vi "TcpDataReceived.vi"(8 "error in (no error)":errorcluster, 10 "DataReceived":refnum<class "DataReceived.lvclass">, 11 "Cli in":refnum<class "Cli.lvclass">) -> (0 "error out":errorcluster, 3 "Cli out":refnum<class "Cli.lvclass">)   [LabVIEW 2022 SP3, in "Cli.lvlib" / "Cli.lvclass"]
uses:
  Cli.lvclass
  Tcp/DataReceived/DataReceived.lvclass
  Cli.lvclass/Cli.ctl
  Tcp/DataReceived/DataReceived.lvclass/DataReceived.ctl
  ArgumentParser/Source/ParsedData/ParsedData.lvclass/ParsedData.ctl
  Tcp/Tcp Messages/ConnectionWriteData Msg/ConnectionWriteData Msg.lvclass/ConnectionWriteData Msg.ctl
  <vilib>/ActorFramework/Message Enqueuer/Message Enqueuer.lvclass/Message Enqueuer.ctl
  Tcp/DataReceived/Read Data.vi
  Tcp/DataReceived/Read Refnum.vi
  ArgumentParser/Source/ParsedData/Read Arguments.vi
  ArgumentParser/Source/ParsedData/Read StdOut.vi
  ArgumentParser/Source/ParsedData/Read StdErr.vi
  <vilib>/ActorFramework/Message Enqueuer/Enqueue.vi
  Tcp/Tcp Messages/ConnectionWriteData Msg/ConnectionWriteData Msg.lvclass
  C:/Program Files (x86)/National Instruments/LabVIEW 2022/vi.lib/ActorFramework/Message/Message.lvclass
  <vilib>/ActorFramework/Message Priority Queue/Priority Enqueue.vi
  ArgumentParser/Source/ArgumentParser/ArgumentParser.lvclass
  Tcp/DataToSend/DataToSend.lvclass
  CommandReceived/CommandReceived.lvclass
  ArgumentParser/Source/ParsedData/ParsedData.lvclass
  <vilib>/ActorFramework/Actor/Actor.lvclass
  CallerMessage Messages/CliCommandReceived Msg/CliCommandReceived Msg.lvclass
  C:/Program Files (x86)/National Instruments/LabVIEW 2022/vi.lib/ActorFramework/Actor/Actor.lvclass
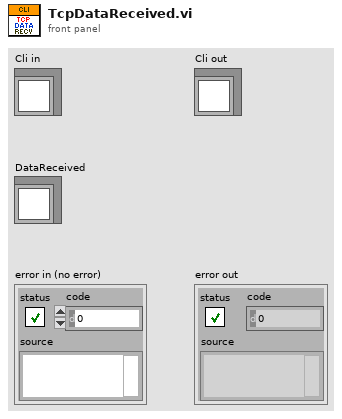
[diagram p1: front panel]
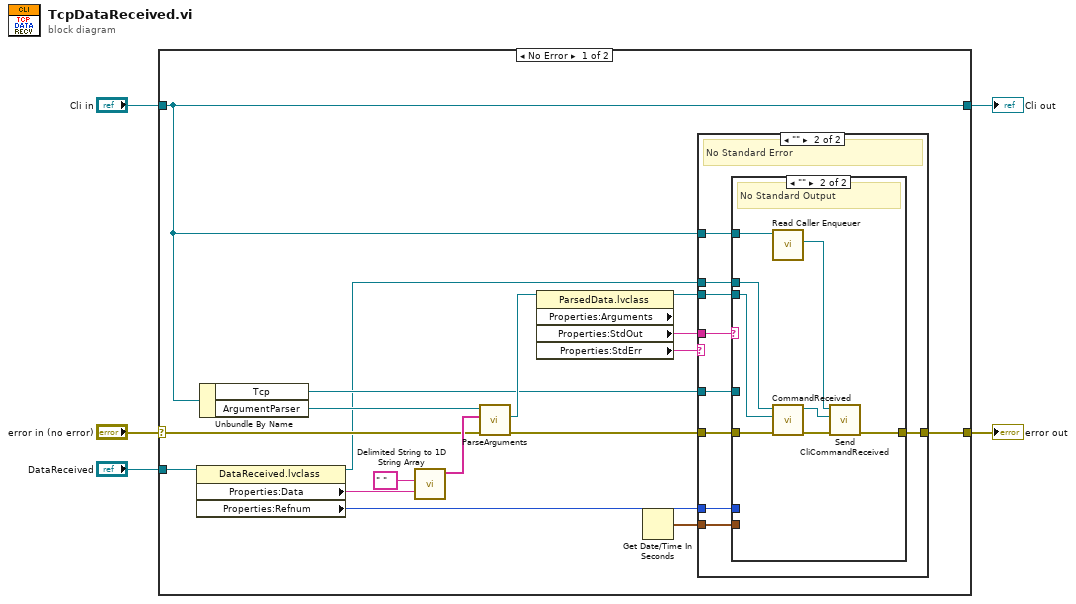
[diagram p0: block diagram]
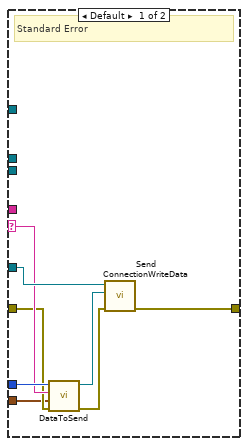
[diagram p2: hidden frame]
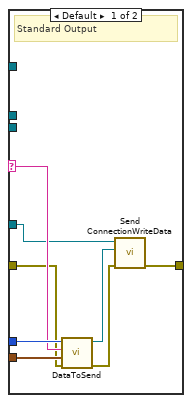
[diagram p3: hidden frame]
diagram:
  n1 = case shown="No Error" "error in (no error)" {
    selector: "error in (no error)" -> [w17 w57]
    tunnel: [w15 w57] -> w2
    tunnel: [w6 w56] -> w1
    tunnel: "Cli in" -> [w6 w56]
    tunnel: "DataReceived" -> [w18 _]
    frame No Error {
      n2 = property class="DataReceived.lvclass"(reference=w18) -> (reference out=w8:refnum<class "DataReceived.lvclass">, "Properties:Data"=w21:string, "Properties:Refnum"=w11:u64)  [unwired: 1 in, 1 out]
      n3 = Unbundle By Name(w6) -> ("Tcp"=w12:refnum<class "Message Enqueuer.lvclass">, "ArgumentParser"=w19:refnum<class "ArgumentParser.lvclass">)
      n4 = call <vilib>:"Delimited String to 1D String Array.vi"("delimiter"=" ", "delimited string"=w21) -> ("string array"=w20:string[])  [unwired: 9 in]
      n5 = call-dynamic "ParseArguments.vi"("error in (no error)"=w17, "CliArguments"=w20, "ArgumentParser in"=w19) -> ("error out"=w14:errorcluster, "ParsedData"=w16:refnum<class "ParsedData.lvclass">)  [unwired: 6 in, 1 out]
      n6 = property class="ParsedData.lvclass" props=["Properties:Arguments", "Properties:StdOut", "Properties:StdErr"](reference=w16) -> (reference out=w7:refnum<class "ParsedData.lvclass">, "Properties:StdOut"=w10:string, "Properties:StdErr"=w13:string)  [unwired: 1 in, 2 out]
      n7 = Get Date/Time In Seconds() -> (seconds since 1Jan1904=w9:timestamp)
      n8 = case shown="\"\"" w13 {
        selector: w13 -> [w27 _]
        tunnel: [w30 w38] -> w15
        tunnel: w14 -> [w25 w37]
        tunnel: w12 -> [w29 w34]
        tunnel: w11 -> [w28 w36]
        tunnel: w10 -> [_ w39]
        tunnel: w9 -> [w23 w35]
        tunnel: w8 -> [_ w33]
        tunnel: w7 -> [_ w32]
        tunnel: w6 -> [_ w31]
        frame Default {
          # "Standard Error"
          n9 = call "DataToSend.vi"("error in (no error)"=w25, "TimeStamp"=w23, "Data"=w27, "Refnum"=w28) -> ("error out"=w26:errorcluster, "DataToSend"=w24:refnum<class "DataToSend.lvclass">)  [unwired: 6 in]
          n10 = call "Send ConnectionWriteData.vi"("error in (no error)"=w26, "DataToSend"=w24, "Message Enqueuer"=w29) -> ("error out"=w30:errorcluster)  [unwired: 7 in, 1 out]
        }
        frame "" {
          # "No Standard Error"
          n11 = case shown="\"\"" w39 {
            selector: w39 -> [w45 _]
            tunnel: [w43 w50] -> w38
            tunnel: w37 -> [w44 w55]
            tunnel: w36 -> [w47 _]
            tunnel: w35 -> [w46 _]
            tunnel: w34 -> [w42 _]
            tunnel: w33 -> [_ w54]
            tunnel: w32 -> [_ w53]
            tunnel: w31 -> [_ w52]
            frame Default {
              # "Standard Output"
              n12 = call "DataToSend.vi"("error in (no error)"=w44, "TimeStamp"=w46, "Data"=w45, "Refnum"=w47) -> ("error out"=w41:errorcluster, "DataToSend"=w40:refnum<class "DataToSend.lvclass">)  [unwired: 6 in]
              n13 = call "Send ConnectionWriteData.vi"("error in (no error)"=w41, "DataToSend"=w40, "Message Enqueuer"=w42) -> ("error out"=w43:errorcluster)  [unwired: 7 in, 1 out]
            }
            frame "" {
              # "No Standard Output"
              n14 = call <vilib>:"Read Caller Enqueuer.vi"("Actor"=w52) -> ("Caller Enqueuer"=w49:refnum<class "Message Enqueuer.lvclass">)  [unwired: 10 in]
              n15 = call "CommandReceived.vi"("error in (no error)"=w55, "ParsedData"=w53, "DataReceived"=w54) -> ("error out"=w51:errorcluster, "CommandReceived"=w48:refnum<class "CommandReceived.lvclass">)  [unwired: 7 in]
              n16 = call "Send CliCommandReceived.vi"("error in (no error)"=w51, "CommandReceived"=w48, "Message Enqueuer"=w49) -> ("error out"=w50:errorcluster)  [unwired: 7 in, 1 out]
            }
          }
        }
      }
    }
    frame Error {
    }
  }
  "error out" <- w2
  "Cli out" <- w1
